vi "Is From Packed Library.vi"(10 "Qualified Name":string) -> (2 "Is From Packed Library":bool)   [LabVIEW 2017, in "Composition.lvlib"]
doc: "Checks if the provided qualified name refers to an interface or class inside a packed library (lvlibp)."
uses:
  Composition.lvlib
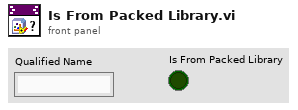
[diagram p1: front panel]
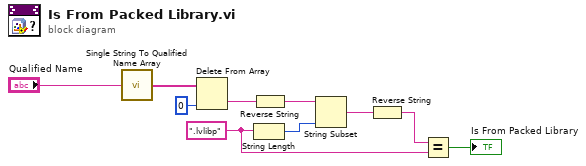
[diagram p0: block diagram]
diagram:
  w4 = ".lvlibp"
  n1 = call <vilib>:"Single String To Qualified Name Array.vi"("Fully Qualified String"="Qualified Name") -> ("Fully Qualified Array"=w3:string[])
  n2 = Delete From Array(array=w3, index=0) -> (deleted portion=w10:string)  [unwired: 1 in, 1 out]
  n3 = String Length(string=w4) -> (length=w7:i32)
  n4 = Reverse String(1:w10) -> (0:w8:string)
  n5 = String Subset(string=w8, length (rest)=w7) -> (substring=w6:string)  [unwired: 1 in]
  n6 = Reverse String(1:w6) -> (0:w5:string)
  n7 = Equal?(x=w5, y=w4) -> (x = y?=→"Is From Packed Library":bool)
